vi "Build Finite Region Array.vi"(10 "Set":set{i32}(c389), 11 "Coordinates":i32[][](array[numeric])) -> (3 "Finite Regions":i32[](array[numeric]))   [LabVIEW 2019]
doc: "Build array of regions that are finite."
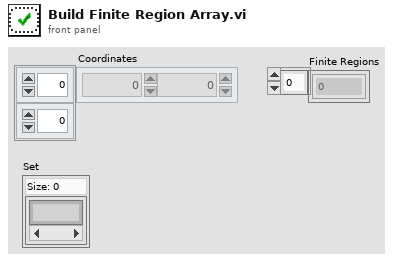
[diagram p1: front panel]
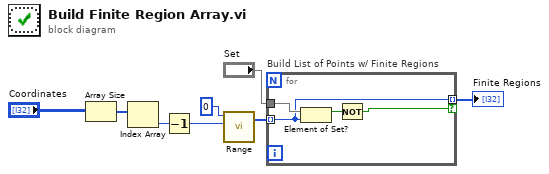
[diagram p0: block diagram]
diagram:
  n1 = Array Size(array="Coordinates") -> (size(s)=w3:i32[])
  n2 = Index Array(array=w3) -> (element=w1:i32)  [unwired: 1 in]
  n3 = Decrement(x=w1) -> (x-1=w7:i32)
  n4 = call "Range.vi"("y"=w7, "x"=0) -> ("Range"=w6:i32[])  [unwired: 5 in]
  n5 = for "Build List of Points w/ Finite Regions" {
    tunnel: "Set" -> [w12]
    tunnel: w6 -> [w11] mode=indexing
    tunnel: [w11] -> w8 mode=indexing if=w9
    n6 = Element of Set?(10:w11, 11:w12) -> (3:w10:bool)
    n7 = Not(x=w10) -> (.not. x?=w9:bool)
  }
  "Finite Regions" <- w8
